vi "Demo1 (Host).vi"() -> ()   [LabVIEW 2023]
uses:
  <vilib>/rvi/interface/nirviOpenFPGA/nirviOpenFPGA.xnode
  <vilib>/rvi/interface/nirviMethod/nirviMethod.xnode
  <vilib>/rvi/interface/nirviCloseFPGA/nirviCloseFPGA.xnode
  <vilib>/addons/Digital Filter Design/NI_DigFilterLicensed.lvlib
  <vilib>/addons/Digital Filter Design/FilterLib.llb/DFD Load MRate Filter from File.vi
  <vilib>/addons/Digital Filter Design/FXPMRateSim.llb/DFD FXP MRate Postprocessing (I16, nCh).vi
  <vilib>/rvi/errors/niLvFpgaMergeErrorWithErrorCode.vi
  FPGA Bitfiles/Demo1_DFDTFilterTarget_Demo1(FPGA)_x49jAZ5l6Bc.lvbitx
  Demo1 (FPGA).vi
  <vilib>/userdefined/High Color/nirio_resource_hc.ctl
panel:
  in  "resource name":T1
  in  "stop":bool
  out "Filtered Signal":dbl[][](graph)
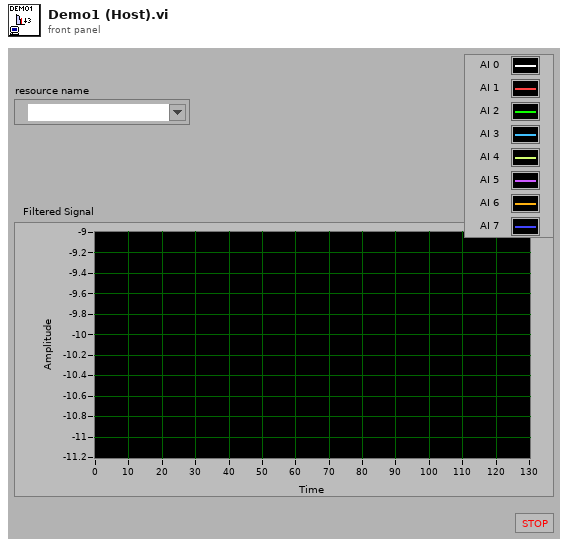
[diagram p1: front panel]
types:
  T1 = typedef "nirio_resource_hc.ctl" = tag
  T2 = typedef "NI_DigFilterLicensed.lvlib/DFD Multirate Filter Obj.ctl" = cluster{"mMRate_Structure":enum16{"CIC", "FIR", "IIR", "Lattice"}, "mMRate_Mode":T3, "mMRate_Factor":i32, "mMRate_FIRParams":cluster{"mMRate_FIR_H":dbl[], "mMRate_FIR_IsNyquist?":bool, "mMRate_FIR_IsSymmetric?":bool}, "mMRate_CICParams":cluster{"mMRate_CIC_#Stage":i32, "mMRate_CIC_Lag":i32, "mMRate_CIC_Type":enum16{"Lowpass", "Highpass"}}, "mMRate_Order":i32, "mMRate_Version":string, "mMRate_Comments":string, "mMRate_RationalFactor":cluster{"mMRate_L":i32, "mMRate_M":i32}, "mMRate_Fs":dbl, "mMRate_Quantized?":bool, "mMRate_QFilterGain":dbl, "mMRate_CoefWl":i16, "mMRate_Scaling":cluster{"mMRate_ScaleByPowerOf2?":bool, "mMRate_ScaleType":T4}, "mMRate_InputWl":i16, "mMRate_OutputWl":i16, "mMRate_OutputMode":T5, "mMRate_MultMode":T6, "mMRate_BitPruning":bool, "mMRate_GainWl":i16, "mMRate_OutputFwl":i16, "mMRate_SumIwl":i16, "mMRate_InputIwl ":i16, "mMRate_SumWl":i16, "mMRate_CoefIwl":i16}
  T3 = typedef "NI_DigFilterLicensed.lvlib/DFD Multirate Mode.ctl" = i16
  T4 = typedef "NI_DigFilterLicensed.lvlib/DFD Coef Norm Type.ctl" = enum16{"No Norm", "Time Domain 1-Norm", "Time Domain 2-Norm", "Time Domain Inf-Norm"}
  T5 = typedef "NI_DigFilterLicensed.lvlib/DFD Round-off Mode.ctl" = enum16{"Nearest", "Truncation"}
  T6 = typedef "NI_DigFilterLicensed.lvlib/DFD FXP MRate Multiply Mode.ctl" = enum16{"Truncated", "Full"}
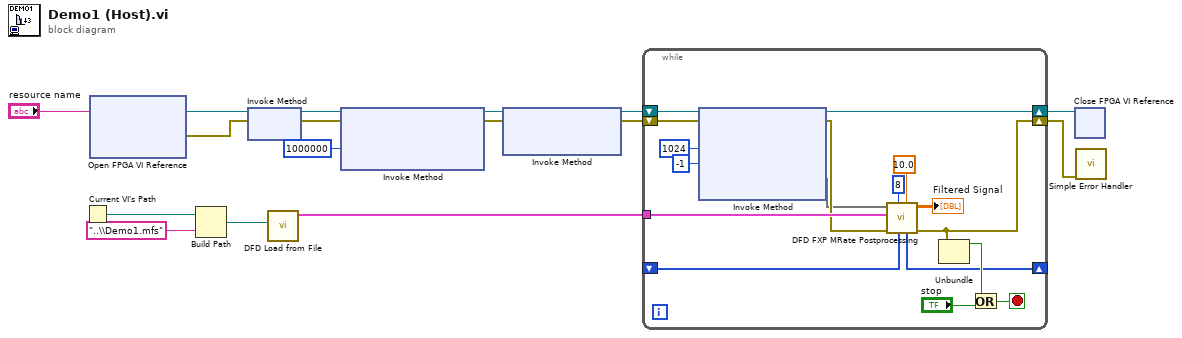
[diagram p0: block diagram]
diagram:
  n1 = Current VI's Path() -> (path=w5:path)
  n2 = xnode "Open FPGA VI Reference"("resource name"="resource name") -> ("FPGA VI Reference Out"=w16:refnum<k20>, "error out"=w15:errorcluster)  [unwired: 1 in]
  n3 = Build Path(base path=w5, name or relative path="..\\Demo1.mfs") -> (appended path=w3:path)
  n4 = xnode "Invoke Method"("FPGA VI Reference In"=w16, "error in"=w15) -> ("FPGA VI Reference Out"=w14:refnum<k20>, "error out"=w13:errorcluster)
  n5 = call-poly <vilib>:"DFD Load from File.vi"("file path in"=w3) -> ("multirate filter out"=w2:T2)  [unwired: 1 in, 9 out]
  n6 = xnode "Invoke Method"("FPGA VI Reference In"=w14, "error in"=w13, "Requested Depth"=u32 1000000 ("Depth")) -> ("FPGA VI Reference Out"=w11:refnum<k20>, "error out"=w10:errorcluster)  [unwired: 1 out]
  n7 = xnode "Invoke Method"("FPGA VI Reference In"=w11, "error in"=w10) -> ("FPGA VI Reference Out"=w9:refnum<k20>, "error out"=w8:errorcluster)  [unwired: 1 in]
  n8 = while {
    shift-right: [w24] -> w6
    shift-left: w8 -> [w32]
    tunnel: w2 -> [w29]
    shift-right: [w25] -> w7
    shift-left: w9 -> [w33]
    shift-right: [w18] -> _
    shift-left: _ -> [w19]
    stop <- w21 stop-if-true
    n9 = xnode "Invoke Method"("FPGA VI Reference In"=w33, "error in"=w32, "Number of Elements"=u32 1024, "Timeout (ms)"=-1) -> ("FPGA VI Reference Out"=w25:refnum<k20>, "error out"=w28:errorcluster, "Data"=w17:void[])  [unwired: 1 out]
    n10 = call-poly <vilib>:"DFD FXP MRate Postprocessing.vi"("input range"=10.0, "history in"=w19, "# channels"=8, "error in (no error)"=w28, "multirate filter"=w29, "signal in"=w17) -> ("error out"=w24:errorcluster, "signal out"=→"Filtered Signal":dbl[][], "history out"=w18:i16[])  [unwired: 3 out]
    n11 = Unbundle(w24) -> ("status"=w22:bool)  [unwired: 2 out]
    n12 = Or(x=w22, y="stop") -> (x .or. y?=w21:bool)
  }
  n13 = xnode "Close FPGA VI Reference"("FPGA VI Reference In"=w7) -> ()  [unwired: 1 in, 1 out]
  n14 = call <vilib>:"Simple Error Handler.vi"("error in (no error)"=w6) -> ()  [unwired: 1 in, 8 out]
